vi "DS18S20 - convert raw temp.vi"(8 "12 Bit?":bool, 10 "Scratchpad Data":u8[](array[numeric])=[0, 0, 0, 0, 0, 0, 0, 0, 0]) -> (2 "Temp (F)":dbl, 3 "Temp (C)":dbl)   [LabVIEW 2012]
panel:
  out "Count per C":u8
  out "Count Remain":u8
  out "MSB":u8 format="%.0x"
  out "LSB":u8 format="%.0x"
  # "Performs the temperature conversion for DS12S20\n- takes the scratchpad data from the device and returns the 9 or 12-bit temp\n- provides temp in C and F"
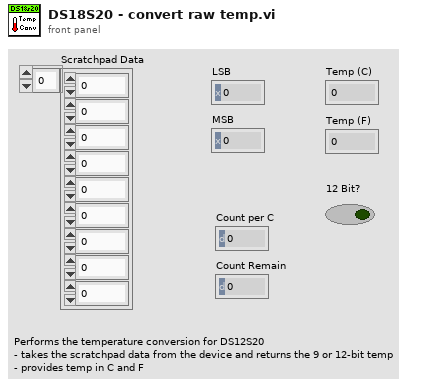
[diagram p1: front panel]
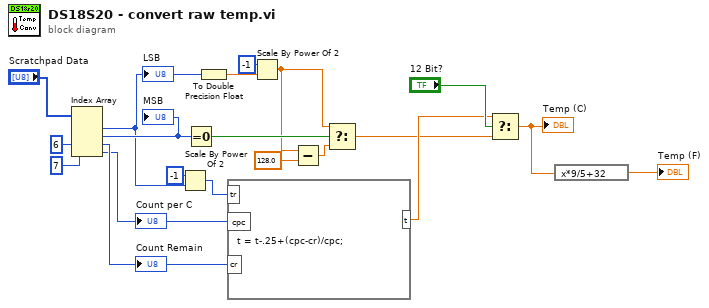
[diagram p0: block diagram]
diagram:
  n1 = Index Array(array="Scratchpad Data", index #3=6 ("index"), index #4=7 ("index")) -> (element #1=w5:u8, element #2=w10:u8, element #3=w9:u8, element #4=w8:u8)  [unwired: 2 in]
  "LSB" <- w5
  "MSB" <- w10
  "Count per C" <- w8
  "Count Remain" <- w9
  n2 = Scale By Power Of 2(n=-1, x=w5) -> (x*2^n=w3:u8)
  n3 = Equal To 0?(x=w10) -> (x = 0?=w18:bool)
  n4 = To Double Precision Float(number=w5) -> (double precision float=w20:dbl)
  n5 = formula code="t = t-.25+(cpc-cr)/cpc;"("cpc"=w8, "cr"=w9, "tr"=w3) -> ("t"=w2:dbl)
  n6 = Scale By Power Of 2(n=-1, x=w20) -> (x*2^n=w17:dbl)
  n7 = Subtract(x=w17, y=128.0) -> (x-y=w16:dbl)
  n8 = Select(t=w17, s=w18, f=w16) -> (s? t:f=w1:dbl)
  n9 = Select(t=w2, s="12 Bit?", f=w1) -> (s? t:f=w7:dbl)
  "Temp (C)" <- w7
  n10 = expression code="x*9/5+32"(w7) -> (→"Temp (F)":dbl)
